vi "subbus_write.vi"(8 "error in (no error)":errorcluster, 9 "PortIn":string, 10 "Data":u16 format="%x", 11 "Address":u16 format="%x") -> (0 "error out":errorcluster, 1 "PortOut":string, 3 "Ack":bool)   [LabVIEW 2016]
uses:
  <vilib>/ErrorRing/Error Ring.xnode
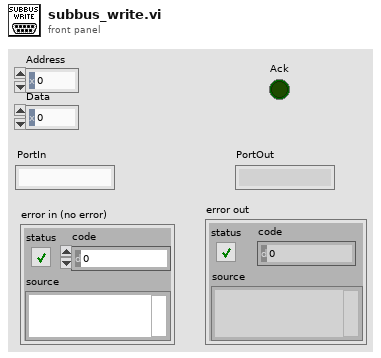
[diagram p1: front panel]
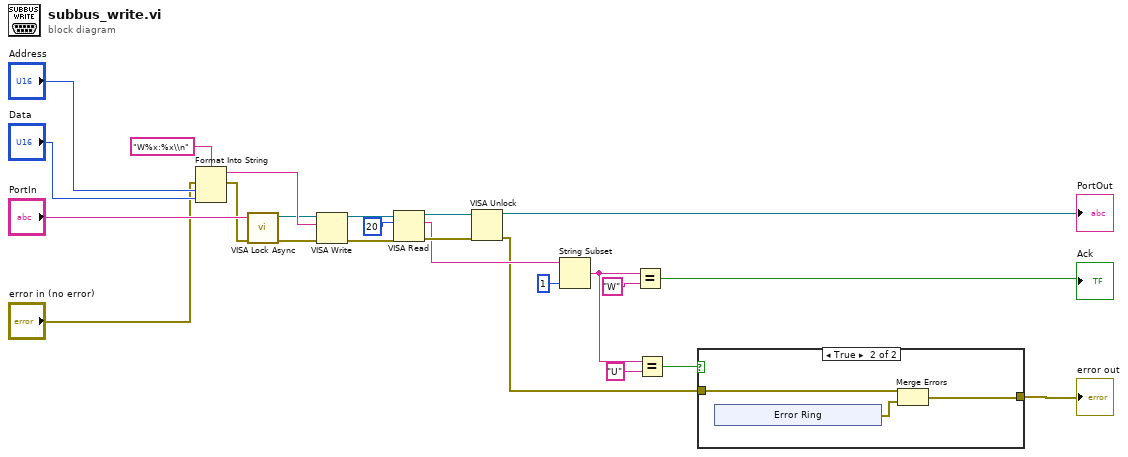
[diagram p0: block diagram]
diagram:
  n1 = Format Into String(format string="W%x:%x\\n", error in="error in (no error)", "Address", "Data") -> (resulting string=w22:string, error out=w2:errorcluster)  [unwired: 1 in]
  n2 = call <vilib>:"VISA Lock Async.vi"("error in (no error)"=w2, "VISA resource name"="PortIn") -> ("error out"=w14:errorcluster, "VISA resource name out"=w15:refnum<visa-resource-name>)  [unwired: 7 in, 1 out]
  n3 = VISA Write(VISA resource name=w15, write buffer=w22, error in (no error)=w14) -> (VISA resource name out=w20:refnum<visa-resource-name>, error out=w21:errorcluster)  [unwired: 1 out]
  n4 = VISA Read(VISA resource name=w20, byte count=20, error in (no error)=w21) -> (VISA resource name out=w18:refnum<visa-resource-name>, read buffer=w11:string, error out=w17:errorcluster)  [unwired: 1 out]
  n5 = VISA Unlock(8:w17, 11:w18) -> (0:w1:errorcluster, 3:→"PortOut":refnum<visa-resource-name>)
  n6 = String Subset(string=w11, length (rest)=1) -> (substring=w9:string)  [unwired: 1 in]
  n7 = Equal?(x=w9, y="W") -> (x = y?=→"Ack":bool)
  n8 = Equal?(x=w9, y="U") -> (x = y?=w7:bool)
  n9 = case shown="True" w7 {
    tunnel: w1 -> [w25 w28]
    tunnel: [w25 w26] -> w6
    frame False {
    }
    frame True {
      n10 = xnode "Error Ring"() -> ("error out"=w27:errorcluster)
      n11 = Merge Errors(w28, w27) -> (w26:errorcluster)
    }
  }
  "error out" <- w6
